vi "OnDataChange.vi"(0 "Microscope in":refnum<class "Microscope.lvclass">, 1 "DataExchange":T1, 3 "error in (no error)":errorcluster) -> (7 "Microscope out":refnum<class "Microscope.lvclass">, 10 "error out":errorcluster)   [LabVIEW 2020, in "Microscope.lvlib" / "Microscope.lvclass"]
uses:
  Microscope.lvclass
  C:/Program Files/National Instruments/LabVIEW 2020/vi.lib/ActorFramework/Actor/Actor.lvclass
  Component/Device/Device/DataExchange.ctl
  <vilib>/vision/Image Controls.llb/IMAQ Image.ctl
  Microscope.lvclass/Microscope.ctl
  Interface/DataListener Messages/OnDataChange Msg/OnDataChange Msg.lvclass/OnDataChange Msg.ctl
  <vilib>/ActorFramework/Message Enqueuer/Message Enqueuer.lvclass/Message Enqueuer.ctl
  <vilib>/ActorFramework/Actor/Actor.lvclass/Actor.ctl
  Hardware Layer/Real Hardware/Camera_Prime95B/Camera_Prime95B/Controls/Camera Status.ctl
  Component/Stage/Stage Messages/SetRelativePositionUm Msg/SetRelativePositionUm Msg.lvclass/SetRelativePositionUm Msg.ctl
  <vilib>/ActorFramework/Message Enqueuer/Enqueue.vi
  Interface/DataListener Messages/OnDataChange Msg/OnDataChange Msg.lvclass
  C:/Program Files/National Instruments/LabVIEW 2020/vi.lib/ActorFramework/Message/Message.lvclass
  Component/Stage/Stage Messages/SetRelativePositionUm Msg/SetRelativePositionUm Msg.lvclass
  <vilib>/ActorFramework/Message Priority Queue/Priority Enqueue.vi
  Interface/DataListener/DataListener.lvclass
  Component/Camera/Camera/Camera.lvclass
  <vilib>/ActorFramework/Actor/Actor.lvclass
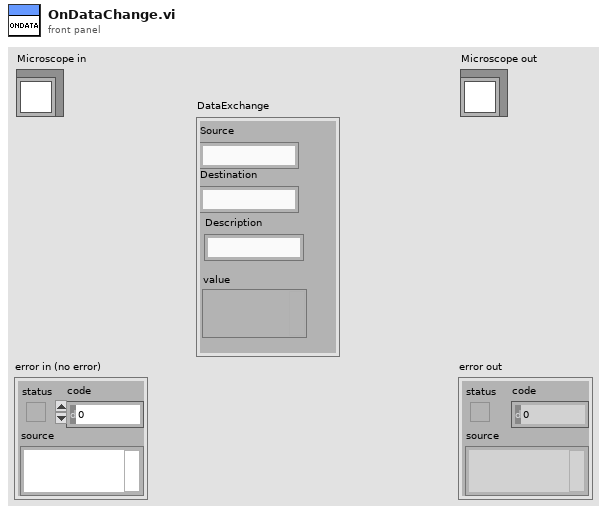
[diagram p1: front panel]
types:
  T1 = typedef "DataListener.lvclass/DataExchange.ctl" = cluster{"Source":string, "Destination":string, "Description":string, "value":variant}
  T2 = typedef "IMAQ Image.ctl" = refnum<image>
  T3 = typedef "Camera.lvlib/Camera.lvclass/Camera Status.ctl" = i32
  T4 = map{string, refnum<class "Message Enqueuer.lvclass">}
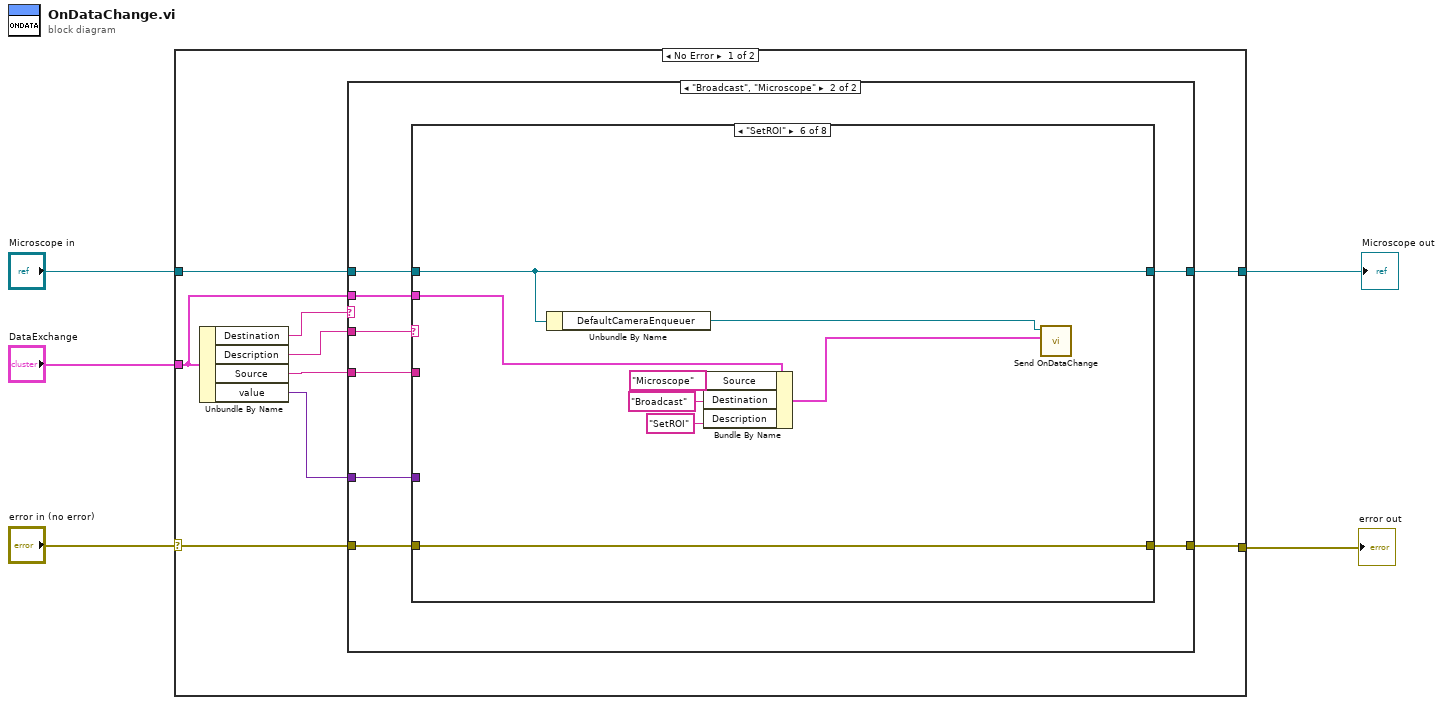
[diagram p0: block diagram]
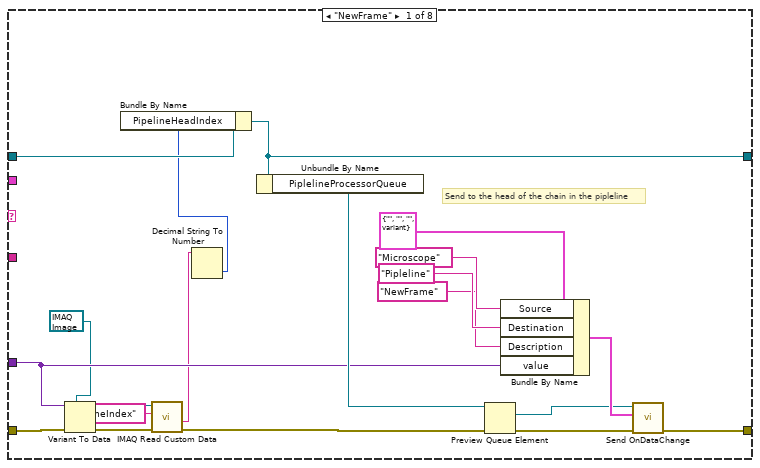
[diagram p3: hidden frame]
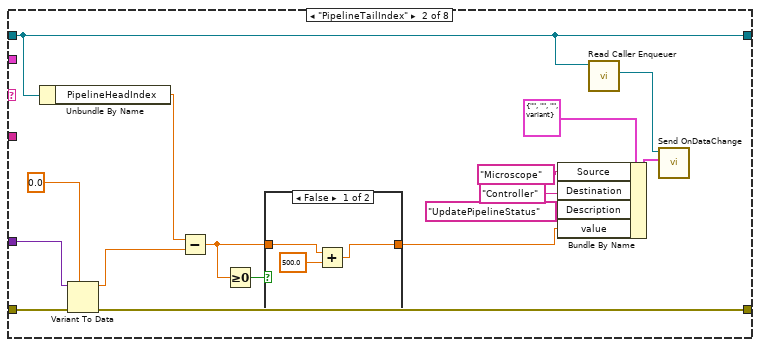
[diagram p4: hidden frame]
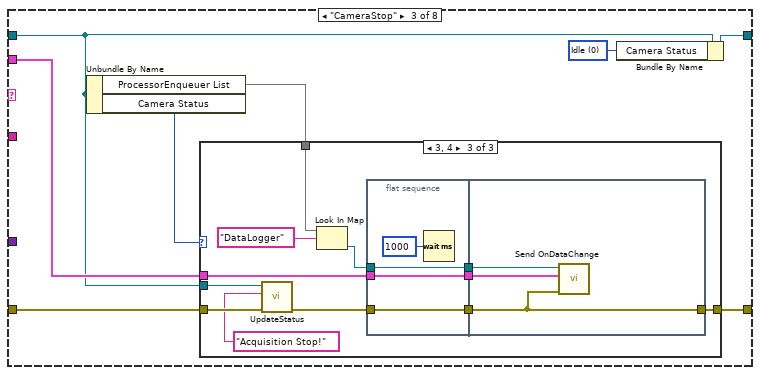
[diagram p6: hidden frame]
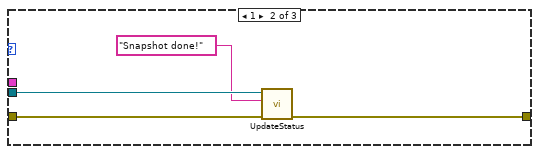
[diagram p8: hidden frame]
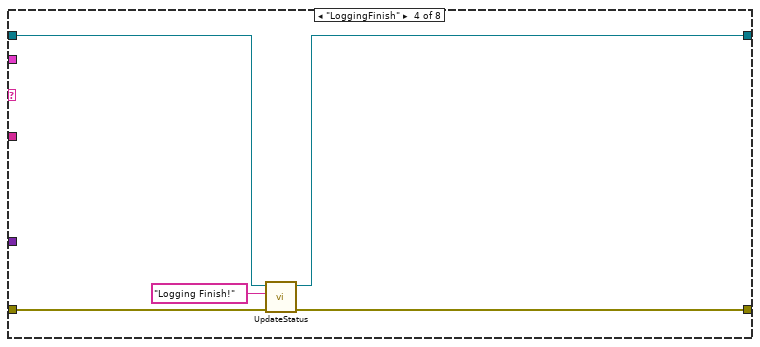
[diagram p9: hidden frame]
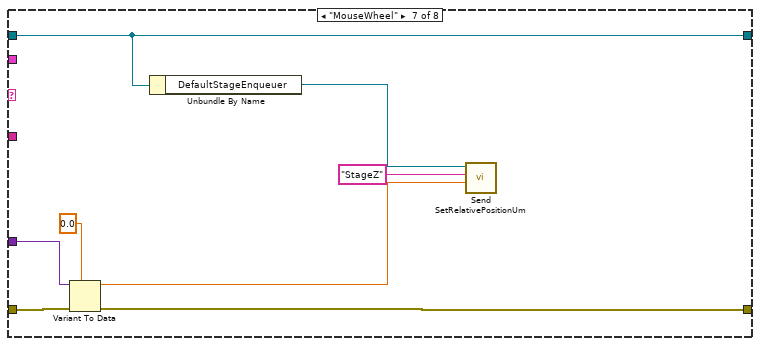
[diagram p11: hidden frame]
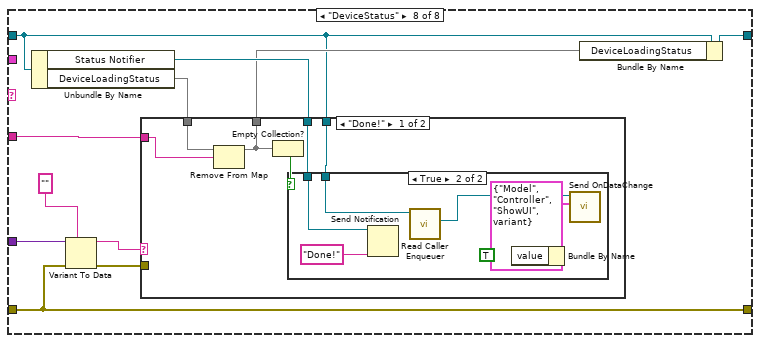
[diagram p12: hidden frame]
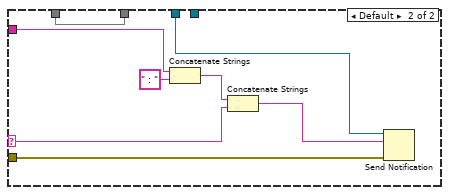
[diagram p14: hidden frame]
diagram:
  n1 = case shown="No Error" "error in (no error)" {
    selector: "error in (no error)" -> [w14 w152]
    tunnel: [w13 w152] -> w4
    tunnel: [w11 w153] -> w2
    tunnel: "Microscope in" -> [w12 w153]
    tunnel: "DataExchange" -> [w6 _]
    frame No Error {
      n2 = Unbundle By Name(w6) -> ("Destination"=w7:string, "Description"=w10:string, "Source"=w8:string, "value"=w9:variant)
      n3 = case shown="\"Broadcast\", \"Microscope\"" w7 {
        tunnel: w14 -> [w15 w24]
        tunnel: [w15 w23] -> w13
        tunnel: w12 -> [w16 w22]
        tunnel: [w16 w21] -> w11
        tunnel: w10 -> [_ w20]
        tunnel: w9 -> [_ w19]
        tunnel: w8 -> [_ w18]
        tunnel: w6 -> [_ w17]
        frame Default {
          # "Ignore all  data that not target/broadcast to microscope"
        }
        frame "Broadcast", "Microscope" {
          n4 = case shown="\"SetROI\"" w20 {
            tunnel: [w41 w59 w69 w100 w102 w111 w118 w129] -> w23
            tunnel: w24 -> [w43 w60 w70 w101 w102 w111 w119 w129]
            tunnel: [w26 w45 w67 w98 w103 w110 w116 w122] -> w21
            tunnel: w22 -> [w44 w45 w68 w99 w103 w110 w116 w120]
            tunnel: w19 -> [w32 w58 _ _ _ _ w117 w127]
            tunnel: w18 -> [_ _ _ _ _ _ _ w123]
            tunnel: w17 -> [_ _ w71 _ _ w104 _ _]
            frame "NewFrame" {
              # "Send to the head of the chain in the pipleline"
              n5 = Variant To Data(error in=w43, type=T2 refnum ("Image Src A"), Variant=w32) -> (data=w29:T2, error out=w33:errorcluster)
              n6 = call "IMAQ Read Custom Data"("error in (no error)"=w33, "Key"="FrameIndex", "Image"=w29) -> ("error out"=w30:errorcluster, "Custom Data Out"=w27:string)  [unwired: 6 in, 1 out]
              n7 = Decimal String To Number(string=w27) -> (number=w25:i32)  [unwired: 2 in, 1 out]
              n8 = Bundle By Name(cluster=w44, "PipelineHeadIndex"=w25) -> (w26:refnum<class "Microscope.lvclass">)
              n9 = Unbundle By Name(w26) -> ("PiplelineProcessorQueue"=w34:refnum<queue>)
              n10 = Preview Queue Element(queue=w34, error in (no error)=w30) -> (element=w35:refnum<class "Message Enqueuer.lvclass">, error out=w42:errorcluster)  [unwired: 1 in, 2 out]
              n11 = Bundle By Name(cluster=T1 {"Source"="", "Destination"="", "Description"="", "value"=variant} ("DataExchange"), "Source"="Microscope", "Destination"="Pipleline", "Description"="NewFrame", "value"=w32) -> (w39:T1)
              n12 = call "Send OnDataChange.vi"("error in (no error)"=w42, "DataExchange"=w39, "Message Enqueuer"=w35) -> ("error out"=w41:errorcluster)  [unwired: 7 in, 1 out]
            }
            frame "PipelineTailIndex" {
              n13 = Unbundle By Name(w45) -> ("PipelineHeadIndex"=w50:dbl)
              n14 = Variant To Data(error in=w60, type=0.0, Variant=w58) -> (data=w49:dbl, error out=w59:errorcluster)
              n15 = Subtract(x=w50, y=w49) -> (x-y=w48:dbl)
              n16 = Greater Or Equal To 0?(x=w48) -> (x >= 0?=w47:bool)
              n17 = case shown="False" w47 {
                tunnel: w48 -> [w63 w64]
                tunnel: [w62 w64] -> w46
                frame False {
                  n18 = Add(x=w63, y=500.0) -> (x+y=w62:dbl)
                }
                frame True {
                }
              }
              n19 = Bundle By Name(cluster=T1 {"Source"="", "Destination"="", "Description"="", "value"=variant} ("DataExchange"), "Source"="Microscope", "Destination"="Controller", "Description"="UpdatePipelineStatus", "value"=w46) -> (w54:T1)
              n20 = call <vilib>:"Read Caller Enqueuer.vi"("Actor"=w45) -> ("Caller Enqueuer"=w56:refnum<class "Message Enqueuer.lvclass">)  [unwired: 10 in]
              n21 = call "Send OnDataChange.vi"("DataExchange"=w54, "Message Enqueuer"=w56) -> ()  [unwired: 8 in, 2 out]
            }
            frame "CameraStop" {
              w65 = T3 0 items=["Idle", "Snap", "Live", "Capturing", "TakeAlbum"] ("Camera Status")
              n22 = Unbundle By Name(w68) -> ("ProcessorEnqueuer List"=w72:T4, "Camera Status"=w66:T3)
              n23 = case shown="3, 4" w66 {
                tunnel: w72 -> [_ _ w86]
                tunnel: w71 -> [_ _ w83]
                tunnel: w70 -> [w73 w77 w82]
                tunnel: [w73 w76 w81] -> w69
                tunnel: w68 -> [_ w75 w79]
                frame 0, Default {
                }
                frame 1 {
                  n24 = call-dynamic "UpdateStatus.vi"("error in (no error)"=w77, "Description"="Snapshot done!", "Microscope in"=w75) -> ("error out"=w76:errorcluster)  [unwired: 7 in, 1 out]
                }
                frame 3, 4 {
                  n25 = call-dynamic "UpdateStatus.vi"("error in (no error)"=w82, "Description"="Acquisition Stop!", "Microscope in"=w79) -> ("error out"=w80:errorcluster)  [unwired: 7 in, 1 out]
                  n26 = Look In Map(map=w86, key="DataLogger") -> (value=w84:refnum<class "Message Enqueuer.lvclass">)  [unwired: 1 in, 1 out]
                  n27 = flat-sequence {
                    tunnel: w80 -> [w91]
                    tunnel: w83 -> [w92]
                    tunnel: w84 -> [w93]
                    tunnel: [w93] -> w89
                    tunnel: [w92] -> w88
                    tunnel: [w91] -> w87
                    tunnel: w89 -> [w96]
                    tunnel: w88 -> [w95]
                    tunnel: w87 -> [w94]
                    tunnel: [w94] -> w81
                    frame #0 {
                      n28 = Wait (ms)(milliseconds to wait=u32 1000) -> ()  [unwired: 1 out]
                    }
                    frame #1 {
                      n29 = call "Send OnDataChange.vi"("error in (no error)"=w94, "DataExchange"=w95, "Message Enqueuer"=w96) -> ()  [unwired: 7 in, 2 out]
                    }
                  }
                }
              }
              n30 = Bundle By Name(cluster=w68, "Camera Status"=w65) -> (w67:refnum<class "Microscope.lvclass">)
            }
            frame "LoggingFinish" {
              n31 = call-dynamic "UpdateStatus.vi"("error in (no error)"=w101, "Description"="Logging Finish!", "Microscope in"=w99) -> ("error out"=w100:errorcluster, "Microscope out"=w98:refnum<class "Microscope.lvclass">)  [unwired: 7 in]
            }
            frame Default {
            }
            frame "SetROI" {
              n32 = Unbundle By Name(w110) -> ("DefaultCameraEnqueuer"=w106:refnum<class "Message Enqueuer.lvclass">)
              n33 = Bundle By Name(cluster=w104, "Source"="Microscope", "Destination"="Broadcast", "Description"="SetROI") -> (w105:T1)
              n34 = call "Send OnDataChange.vi"("DataExchange"=w105, "Message Enqueuer"=w106) -> ()  [unwired: 8 in, 2 out]
            }
            frame "MouseWheel" {
              n35 = Variant To Data(error in=w119, type=0.0 ("height"), Variant=w117) -> (data=w112:dbl, error out=w118:errorcluster)
              n36 = Unbundle By Name(w116) -> ("DefaultStageEnqueuer"=w114:refnum<class "Message Enqueuer.lvclass">)
              n37 = call "Send SetRelativePositionUm.vi"("RelativeMoveum"=w112, "Stage Label"="StageZ", "Message Enqueuer"=w114) -> ()  [unwired: 7 in, 2 out]
            }
            frame "DeviceStatus" {
              n38 = Unbundle By Name(w120) -> ("Status Notifier"=w130:refnum<notifier>, "DeviceLoadingStatus"=w124:map{string, bool})
              n39 = Variant To Data(error in=w129, type="" ("notification"), Variant=w127) -> (data=w125:string, error out=w126:errorcluster)
              n40 = case shown="\"Done!\"" w125 {
                selector: w125 -> [_ w144]
                tunnel: w130 -> [w136 w151]
                tunnel: w126 -> [_ w150]
                tunnel: w124 -> [w135 w149]
                tunnel: w123 -> [w134 w148]
                tunnel: [w132 w149] -> w121
                tunnel: w120 -> [w131 _]
                frame "Done!" {
                  n41 = Remove From Map(10:w134, 11:w135) -> (3:w132:map{string, bool})  [unwired: 2 out]
                  n42 = Empty Collection?(1:w132) -> (0:w133:bool)
                  n43 = case shown="True" w133 {
                    tunnel: w136 -> [_ w143]
                    tunnel: w131 -> [_ w141]
                    frame False {
                    }
                    frame True {
                      n44 = Send Notification(notification="Done!", notifier=w143) -> ()  [unwired: 1 in, 2 out]
                      n45 = call <vilib>:"Read Caller Enqueuer.vi"("Actor"=w141) -> ("Caller Enqueuer"=w137:refnum<class "Message Enqueuer.lvclass">)  [unwired: 10 in]
                      n46 = Bundle By Name(cluster=T1 {"Source"="Model", "Destination"="Controller", "Description"="ShowUI", "value"=variant} ("DataExchange"), "value"=TRUE) -> (w139:T1)
                      n47 = call "Send OnDataChange.vi"("DataExchange"=w139, "Message Enqueuer"=w137) -> ()  [unwired: 8 in, 2 out]
                    }
                  }
                }
                frame Default {
                  n48 = Concatenate Strings(w148, " : " ("string")) -> (w146:string)
                  n49 = Concatenate Strings(w146, w144) -> (w145:string)
                  n50 = Send Notification(notification=w145, notifier=w151, error in (no error)=w150) -> ()  [unwired: 2 out]
                }
              }
              n51 = Bundle By Name(cluster=w120, "DeviceLoadingStatus"=w121) -> (w122:refnum<class "Microscope.lvclass">)
            }
          }
        }
      }
    }
    frame Error {
    }
  }
  "error out" <- w4
  "Microscope out" <- w2
